vi "NI 9230 Getting Started (Host).vi"() -> ()   [LabVIEW 2021]
doc: "This VI runs on the host device. The host can be a Windows PC or Real-Time target. The example reads a buffer of single point values from all three channels of the NI 9232."
uses:
  <vilib>/userDefined/High Color/nirio_resource_hc.ctl
  <vilib>/LabVIEW Targets/FPGA/cRIO/shared/nicrio_ModuleControls/nicrio_cRIO-9232_ConfigModeRing.ctl
  <vilib>/LabVIEW Targets/FPGA/cRIO/shared/nicrio_ModuleControls/nicrio_cRIO-9230_DataRatesRing2.ctl
  <vilib>/FPGAPlugInAG/cRIO-9053/niLvFpga_Open_cRIO-9053.vi
  <vilib>/rvi/interface/common/dynamic/niFpgaDynamicAddResources.vi
  <vilib>/FPGAPlugInAG/Dynamic/niLvFpga_Reset_Dynamic.vi
  <vilib>/Utility/error.llb/Error Cluster From Error Code.vi
  <vilib>/rvi/errors/niLvFpgaAdjustHostInterfaceError.vi
  <vilib>/FPGAPlugInAG/Dynamic/niLvFpga_Run_Dynamic.vi
  <vilib>/RVI Host/nirviSupport.llb/nirviErrorClusterFromErrorCode.vi
  <vilib>/LabVIEW Targets/FPGA/RIO/CompactRIO/cRIO-91xx/cRIO-91XX_ReadTEDSImpl.vi
  <vilib>/FPGAPlugInAG/Dynamic/niLvFpga_Close_Dynamic.vi
  <vilib>/rvi/interface/nirviOpenFPGA/nirviOpenFPGA.xnode
  FPGA Bitfiles/ni9230gettingsta_FPGATarget2_NI9230GettingSta_c6zQ8chLpPs.lvbitx
  NI 9230 Getting Started (FPGA).vi
  <vilib>/rvi/interface/nirviMethod/nirviMethod.xnode
  <vilib>/rvi/interface/nirviReadWriteControl/nirviReadWriteControl.xnode
  <vilib>/rvi/interface/nirviCloseFPGA/nirviCloseFPGA.xnode
  <vilib>/rvi/interface/Simulation/niFpgaSimulationCallBeginRW.vi
  <vilib>/rvi/interface/nirviMethod/StockFPGA_InlinedMethodWaitForSingleIRQ.vi
  <vilib>/FPGAPlugInAG/Dynamic/niLvFpga_WaitOnIrq_Dynamic.vi
  <vilib>/FPGAPlugInAG/Dynamic/niLvFpga_AcknowledgeIrq_Dynamic.vi
  <vilib>/FPGAPlugInAG/Dynamic/niLvFpga_ReadFifo_Dynamic.vi
  <vilib>/rvi/errors/niLvFpgaMergeErrorWithErrorCode.vi
  NiFpgaLv.dll
panel:
  out "XY Graph":cluster{dbl[], dbl[]}(graph)
  out "Waveform Graph 3":waveform(dbl)(graph)={"t0"=timestamp(0 s since 1904-01-01), "dt"=0.0009765625, "Y"=array[511 elements]}
  out "Waveform Graph 2":waveform(dbl)(graph)={"t0"=timestamp(0 s since 1904-01-01), "dt"=0.0009765625, "Y"=array[511 elements]}
  in  "Input Configuration 2":T1=1 items=["AC Coupled", "DC Coupled", "IEPE AC Coupled"]
  in  "Input Configuration 1":T1=1 items=["AC Coupled", "DC Coupled", "IEPE AC Coupled"]
  in  "Save data":bool caption="Enable"
  in  "Filename":path=path "C:/Users/data/2023_03_10_data_2-out1_out3_in2.lvm"
  in  "Host Loop update rate (ms)":u32=500
  in  "Data Rate":T2=102 items=["12.800 kS/s (NI 9230)"=10, "11.378 kS/s (NI 9230)"=36, "10.240 kS/s (NI 9230)"=21, "9.309 kS/s (NI 9230)"=44, "8.533 kS/s (NI 9230)"=14, "7.877 kS/s (NI 9230)"=52, "7.314 kS/s (NI 9230)"=29, "6.827 kS/s (NI 9230)"=60, "6.400 kS/s (NI 9230)"=18, "6.024 kS/s (NI 9230)"=68, "5.689 kS/s (NI 9230)"=37, "5.389 kS/s (NI 9230)"=76, "5.120 kS/s (NI 9230)"=22, "4.876 kS/s (NI 9230)"=84, "4.655 kS/s (NI 9230)"=45, "4.452 kS/s (NI 9230)"=92, "4.267 kS/s (NI 9230)"=26, "4.096 kS/s (NI 9230)"=100, "3.938 kS/s (NI 9230)"=53, "3.657 kS/s (NI 9230)"=30, "3.413 kS/s (NI 9230)"=61, "3.200 kS/s (NI 9230)"=34, "3.012 kS/s (NI 9230)"=69, "2.844 kS/s (NI 9230)"=38, "2.695 kS/s (NI 9230)"=77, "2.560 kS/s (NI 9230)"=42, "2.438 kS/s (NI 9230)"=85, "2.327 kS/s (NI 9230)"=46, "2.226 kS/s (NI 9230)"=93, "2.133 kS/s (NI 9230)"=50, "2.048 kS/s (NI 9230)"=101, "1.969 kS/s (NI 9230)"=54, "1.829 kS/s (NI 9230)"=58, "1.707 kS/s (NI 9230)"=62, "1.600 kS/s (NI 9230)"=66, "1.506 kS/s (NI 9230)"=70, "1.422 kS/s (NI 9230)"=74, "1.347 kS/s (NI 9230)"=78, "1.280 kS/s (NI 9230)"=82, "1.219 kS/s (NI 9230)"=86, "1.164 kS/s (NI 9230)"=90, "1.113 kS/s (NI 9230)"=94, "1.067 kS/s (NI 9230)"=98, "1.024 kS/s (NI 9230)"=102, "0.985 kS/s (NI 9230)"=106]
  in  "stop":bool
  out "Elements Remaining":u32
  out "FPGA error out":errorcluster
  out "Host error out":errorcluster
  out "Open Loop":bool[](array[boolean])
  out "Short Circuit":bool[](array[boolean])
  out "Data FIFO Full":bool
  in  "Input Configuration 0":T1=1 items=["AC Coupled", "DC Coupled", "IEPE AC Coupled"]
  in  "TEDS Template File Directory":path=path "C:/"
  in  "Display TEDS Data":bool
  in  "RIO Device":T3="RIO0"
  out "Waveform Graph":waveform(dbl)(graph)={"t0"=timestamp(0 s since 1904-01-01), "dt"=0.0009765625, "Y"=array[511 elements]}
  # "Overview: Demonstrates how to acquire data from the NI 9230\nRequirements: LabVIEW Full Development System, LV FPGA, and NI RIO\nInstructions: \n1. Run this VI."
  # "Resource Parameters"
  # "Timing Parameters"
  # "Ch0"
  # "Ch1"
  # "Ch2"
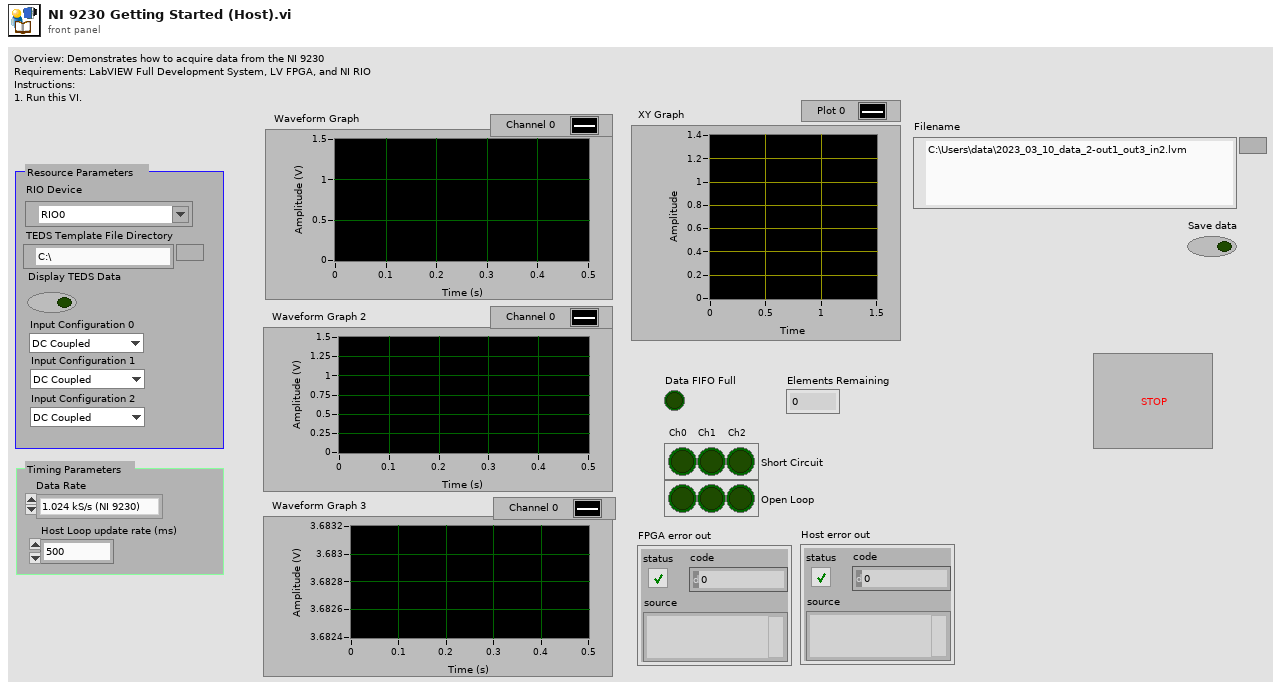
[diagram p1: front panel]
types:
  T1 = typedef "nicrio_cRIO-9232_ConfigModeRing.ctl" = u8
  T2 = typedef "nicrio_cRIO-9230_DataRatesRing2.ctl" = u8
  T3 = typedef "nirio_resource_hc.ctl" = tag
  T4 = cluster{"TEDS Error?":bool, "TEDS Error":string, "TEDS Data":string[][]}
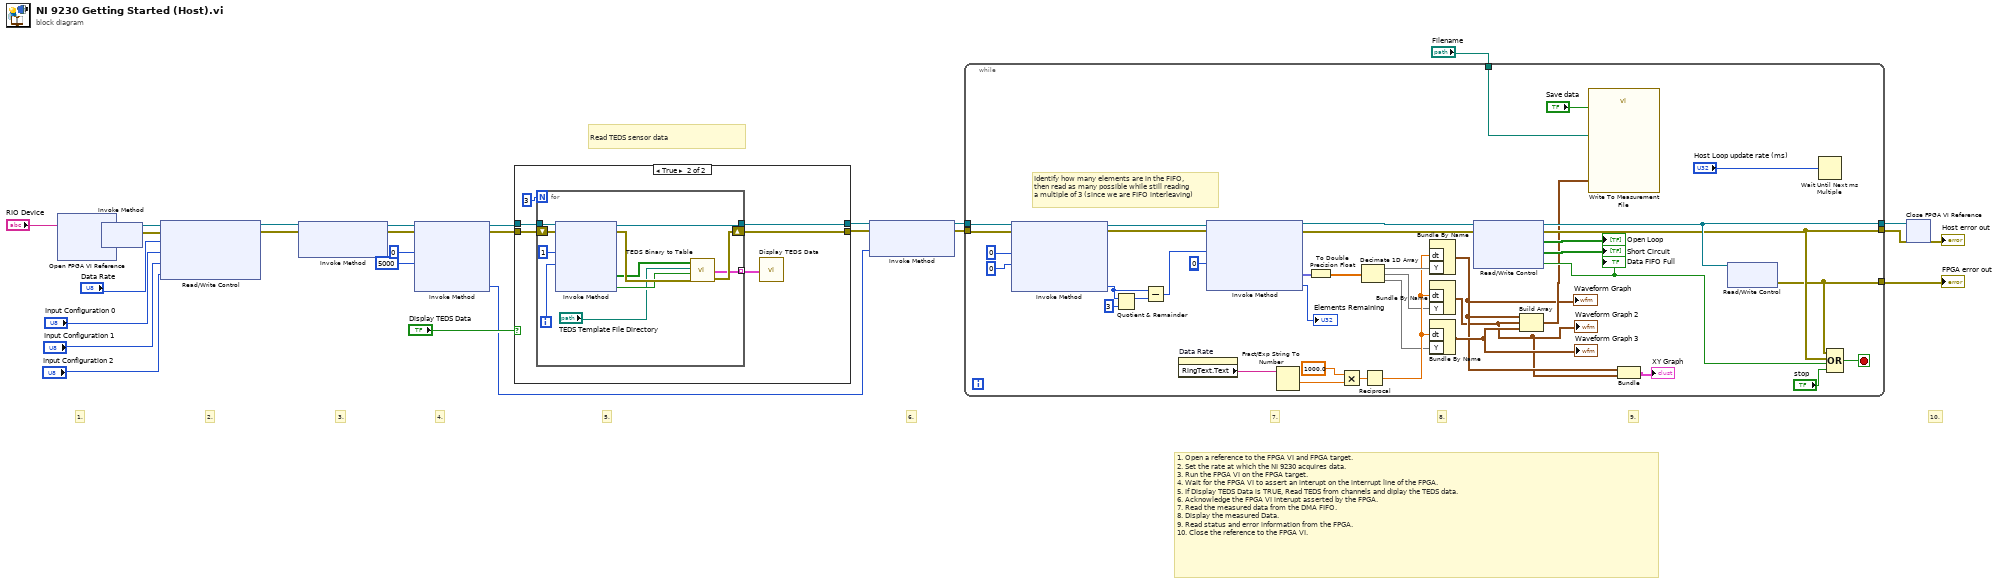
[diagram p0: block diagram]
diagram:
  # "10."
  # "8."
  # "9."
  # "7."
  # "6."
  # "5."
  # "3."
  # "4."
  # "2."
  # "1."
  # "1. Open a reference to the FPGA VI and FPGA target.\n2. Set the rate at which the NI 9230 acquires data.  \n3. Run the FPGA VI on the FPGA target. \n4. Wait for the FPGA VI to assert an interupt on the interrupt line of the FPGA.\n5. If Display TEDS Data is TRUE, Read TEDS from channels and diplay the TEDS data.\n6. Acknowledge the FPGA VI interupt asserted by the FPGA.\n7. Read the measured data from the DMA FIFO.\n8. Display the measured Data.\n9. Read status and error information from the FPGA.\n10. Close the reference to the FPGA VI."
  # "Read TEDS sensor data"
  n1 = xnode "Open FPGA VI Reference"("resource name"="RIO Device") -> ("FPGA VI Reference Out"=w8:refnum<k20>, "error out"=w16:errorcluster)  [unwired: 1 in]
  n2 = xnode "Invoke Method"("FPGA VI Reference In"=w8, "error in"=w16) -> ("FPGA VI Reference Out"=w7:refnum<k20>, "error out"=w9:errorcluster)
  n3 = xnode "Read/Write Control"("FPGA VI Reference In"=w7, "error in"=w9, "Data Rate"="Data Rate", "Input Configuration 0"="Input Configuration 0", "Input Configuration 1"="Input Configuration 1", "Input Configuration 2"="Input Configuration 2") -> ("FPGA VI Reference Out"=w20:refnum<k20>, "error out"=w19:errorcluster)
  n4 = xnode "Invoke Method"("FPGA VI Reference In"=w20, "error in"=w19) -> ("FPGA VI Reference Out"=w18:refnum<k20>, "error out"=w17:errorcluster)  [unwired: 1 in]
  n5 = xnode "Invoke Method"("FPGA VI Reference In"=w18, "error in"=w17, "IRQ Number(s)"=0, "Timeout (ms)"=5000 ("Timeout")) -> ("FPGA VI Reference Out"=w25:refnum<k20>, "error out"=w24:errorcluster, "IRQ(s) Asserted"=w21:i32)  [unwired: 1 out]
  n6 = case shown="True" "Display TEDS Data" {
    tunnel: w25 -> [w30 w36]
    tunnel: [w30 w35] -> w23
    tunnel: w24 -> [w29 w34]
    tunnel: [w29 w31] -> w22
    frame False {
    }
    frame True {
      n7 = for {
        N: 3 -> [_]
        tunnel: w36 -> [w47]
        tunnel: [w46] -> w35
        tunnel: [w41] -> w32 mode=indexing
        shift-right: [w42] -> w31
        shift-left: w34 -> [w45]
        i -> [w40]
        n8 = xnode "Invoke Method"("FPGA VI Reference In"=w47, "error in"=w45, "Slot"=1, "Channel"=w40) -> ("FPGA VI Reference Out"=w46:refnum<k20>, "error out"=w43:errorcluster, "TEDS Binary"=w38:bool[], "v0.9 (TEDS)"=w39:bool)
        n9 = call "TEDS Binary to Table.vi"("error in"=w43, "v0.9 TEDS (F)"=w39, "template file directory"="TEDS Template File Directory", "TEDS Binary"=w38) -> ("error out"=w42:errorcluster, "TEDS"=w41:T4)  [unwired: 1 out]
      }
      n10 = call "Display TEDS Data.vi"("TEDS Array"=w32) -> ()  [unwired: 4 out]
    }
  }
  n11 = xnode "Invoke Method"("FPGA VI Reference In"=w23, "error in"=w22, "IRQ Number(s)"=w21) -> ("FPGA VI Reference Out"=w13:refnum<k20>, "error out"=w12:errorcluster)
  n12 = while {
    tunnel: [w71] -> w10
    tunnel: [w70] -> w15
    tunnel: w13 -> [w61]
    tunnel: w12 -> [w60]
    tunnel: [w69] -> w6
    tunnel: "Filename" -> [w56]
    stop <- w87 stop-if-true
    (unwired) 0 ("Timeout (ms)")
    # "Identify how many elements are in the FIFO, \nthen read as many possible while still reading\na multiple of 3 (since we are FIFO interleaving)"
    n13 = xnode "Invoke Method"("FPGA VI Reference In"=w61, "error in"=w60, "Number of Elements"=u32 0, "Timeout (ms)"=0) -> ("FPGA VI Reference Out"=w63:refnum<k20>, "error out"=w62:errorcluster, "Elements Remaining"=w68:u32)  [unwired: 1 out]
    n14 = Quotient & Remainder(x=w68, y=u32 3) -> (x-y*floor(x/y)=w67:u32)  [unwired: 1 out]
    n15 = Subtract(x=w68, y=w67) -> (x-y=w64:u32)
    n16 = property on="Data Rate" class="Ring (strict)"() -> ("RingText.Text"=w58:string)  [unwired: 2 in, 2 out]
    n17 = xnode "Invoke Method"("FPGA VI Reference In"=w63, "error in"=w62, "Number of Elements"=w64, "Timeout (ms)"=0 ("Timeout")) -> ("FPGA VI Reference Out"=w82:refnum<k20>, "error out"=w81:errorcluster, "Data"=w78:fxp<+/-,24,7>[], "Elements Remaining"=→"Elements Remaining":u32)
    n18 = Fract/Exp String To Number(string=w58) -> (number=w86:dbl)  [unwired: 4 out]
    n19 = To Double Precision Float(number=w78) -> (double precision float=w77:dbl[])
    n20 = Multiply(x=1000.0, y=w86) -> (x*y=w85:dbl)
    n21 = Decimate 1D Array(w77) -> (w83:dbl[], w52:dbl[], w51:dbl[])
    n22 = Reciprocal(x=w85) -> (1/x=w79:dbl)
    n23 = Bundle By Name("dt"=w79, "Y"=w83) -> (w50:waveform(dbl))  [unwired: 1 out]
    "Waveform Graph" <- w50
    n24 = Bundle By Name("dt"=w79, "Y"=w52) -> (w49:waveform(dbl))  [unwired: 1 out]
    "Waveform Graph 2" <- w49
    n25 = Bundle By Name("dt"=w79, "Y"=w51) -> (w53:waveform(dbl))  [unwired: 1 out]
    "Waveform Graph 3" <- w53
    n26 = xnode "Read/Write Control"("FPGA VI Reference In"=w82, "error in"=w81) -> ("FPGA VI Reference Out"=w71:refnum<k20>, "error out"=w70:errorcluster, "Open Loop"=→"Open Loop":bool[], "Short Circuit"=→"Short Circuit":bool[], "Data FIFO Full"=w74:bool)
    "Data FIFO Full" <- w74
    n27 = Build Array(w50, w49, w53) -> (w55:waveform(dbl)[])
    n28 = call "Write To Measurement File"("Signals"=w55, "Enable"="Save data", "Filename"=w56) -> ()  [unwired: 14 in, 3 out]
    n29 = Bundle(w50, w49) -> (→"XY Graph":cluster{waveform(dbl), waveform(dbl)})  [unwired: 1 in]
    n30 = xnode "Read/Write Control"("FPGA VI Reference In"=w71) -> ("Error Out"=w69:errorcluster)  [unwired: 1 in, 2 out]
    n31 = Wait Until Next ms Multiple(millisecond multiple="Host Loop update rate (ms)") -> ()  [unwired: 1 out]
    n32 = Compound Arithmetic op=OR(w69, w70, w74, "stop") -> (w87:bool)
  }
  "FPGA error out" <- w6
  n33 = xnode "Close FPGA VI Reference"("FPGA VI Reference In"=w10, "error in"=w15) -> ("error out"=→"Host error out":errorcluster)
